vi "WriteINI.vi"(0 "ButtonEnum":T1=enum."Middle Button", 11 "error in":errorcluster) -> (15 "error out":errorcluster)   [LabVIEW 2020]
uses:
  ButtonDialogEnum.ctl
  <vilib>/Utility/config.llb/Write Key (String).vi
  <vilib>/Utility/config.llb/NI_LVConfig.lvlib
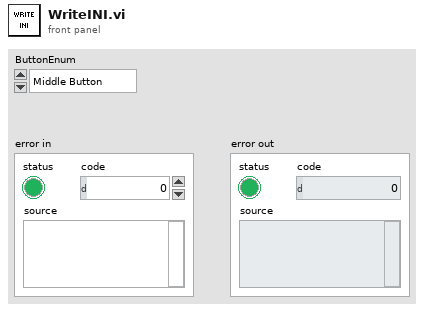
[diagram p1: front panel]
types:
  T1 = typedef "ButtonDialogEnum.ctl" = enum16{"Left Button", "Middle Button", "Right Button", "Window Close"}
  T2 = typedef "NI_LVConfig.lvlib/Config Data RefNum.ctl" = refnum<k1>
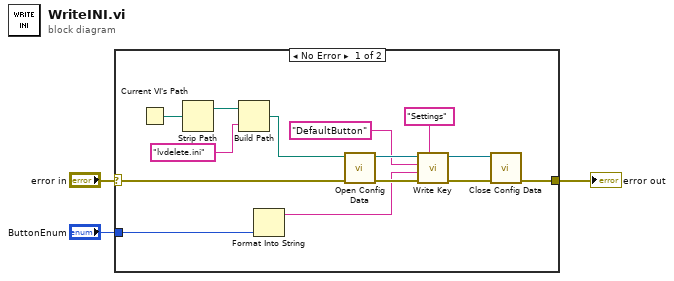
[diagram p0: block diagram]
diagram:
  n1 = case shown="No Error" "error in" {
    selector: "error in" -> [w10 w18]
    tunnel: [w9 w18] -> w2
    tunnel: "ButtonEnum" -> [w5 _]
    frame No Error {
      n2 = Current VI's Path() -> (path=w17:path)
      n3 = Strip Path(path=w17) -> (stripped path=w16:path)  [unwired: 1 out]
      n4 = Build Path(base path=w16, name or relative path="lvdelete.ini") -> (appended path=w8:path)
      n5 = Format Into String(w5) -> (resulting string=w4:string)  [unwired: 3 in, 1 out]
      n6 = call <vilib>:"Open Config Data.vi"("error in (no error)"=w10, "configuration file path"=w8) -> ("error out"=w12:errorcluster, "refnum"=w13:T2)  [unwired: 7 in, 1 out]
      n7 = call-poly <vilib>:"Write Key.vi"("section"="Settings", "error in (no error)"=w12, "value"=w4, "key"="DefaultButton", "refnum"=w13) -> ("error out"=w11:errorcluster, "refnum out"=w14:T2)  [unwired: 4 in, 1 out]
      n8 = call <vilib>:"Close Config Data.vi"("error in (no error)"=w11, "refnum"=w14) -> ("error out"=w9:errorcluster)  [unwired: 8 in, 1 out]
    }
    frame Error {
    }
  }
  "error out" <- w2
